vi "chooseXMLInstantiation.vi"(8 "error in (no error)":errorcluster, 10 "XMLin":string, 11 "TCSTcsCommand in":refnum<class "TCSTcsCommand.lvclass">) -> (0 "error out":errorcluster, 3 "TCSTcsCommand out":refnum<class "TCSTcsCommand.lvclass">)   [LabVIEW 2022 SP3, in "TCSDataDefinitions.lvlib" / "TCSCommand.lvlib" / "TCSTcsCommand.lvclass"]
uses:
  TCSTcsCommand.lvclass
  TCSCommand/commandInstantiation.ctl
  InstrumentSelect/InstrumentSelect.lvclass
  C:/Development/rimas/RIMAS/TCS/TCS_external_interfaces/TCSDataDefinitions/TCSCommand/TCSTcsCommand/TCSTcsCommand.lvclass
  TCSDebug/TCSDebug.lvclass
  M1Cover/M1Cover.lvclass
  OffsetCommands/ScienceTargetOffset/ScienceTargetOffset.lvclass
  OffsetCommands/GuideTargetOffset/GuideTargetOffset.lvclass
  OffsetCommands/WavefrontTargetOffset/WavefrontTargetOffset.lvclass
  OffsetCommands/ScienceTargetAbsorbOffset/ScienceTargetAbsorbOffset.lvclass
  OffsetCommands/GuideTargetAbsorbOffset/GuideTargetAbsorbOffset.lvclass
  OffsetCommands/WavefrontAbsorbOffset/WavefrontAbsorbOffset.lvclass
  OffsetCommands/ScienceTargetClearOffset/ScienceTargetClearOffset.lvclass
  OffsetCommands/GuideTargetClearOffset/GuideTargetClearOffset.lvclass
  OffsetCommands/WavefrontTargetClearOffset/WavefrontTargetClearOffset.lvclass
  OffsetCommands/ClearCollOffset/ClearCollOffset.lvclass
  OffsetCommands/CollOffset/CollOffset.lvclass
  OffsetCommands/RotOffset/RotOffset.lvclass
  POriginCommands/POrigin/POrigin.lvclass
  POriginCommands/POffset/POffset.lvclass
  POriginCommands/AbsorbPOrigin/AbsorbPOrigin.lvclass
  POriginCommands/ClearPOrigin/ClearPOrigin.lvclass
  AmLimit/AmLimit.lvclass
  SetAccessMode/SetOperatorAccessMode/SetOperatorAccessMode.lvclass
  SetAccessMode/SetEngineerAccessMode/SetEngineerAccessMode.lvclass
  StartUp/StartUp.lvclass
  ShutDown/ShutDown.lvclass
  GuiderCommands/Guide/Guide.lvclass
  GuiderCommands/GuideClear/GuideClear.lvclass
  GuiderCommands/GuideAutoclearState/GuideAutoclearState.lvclass
  PointingFileCommands/PointNew/PointNew.lvclass
  PointingFileCommands/PointAdd/PointAdd.lvclass
  TargetConfiguration/WavefrontTargetConfiguration/WavefrontTargetConfiguration.lvclass
  TargetConfiguration/GuideTargetConfiguration/GuideTargetConfiguration.lvclass
  TargetConfiguration/ScienceTargetConfiguration/ScienceTargetConfiguration.lvclass
  CableWrapCommands/RotCurrentWrap/RotCurrentWrap.lvclass
  CableWrapCommands/AzCurrentWrap/AzCurrentWrap.lvclass
  <vilib>/Utility/error.llb/Trim Whitespace.vi
  <vilib>/Utility/error.llb/Trim Whitespace One-Sided.vi
  <userlib>/Common/XML/XMLParser/XMLParser.lvclass
  TCSCommand.lvlib
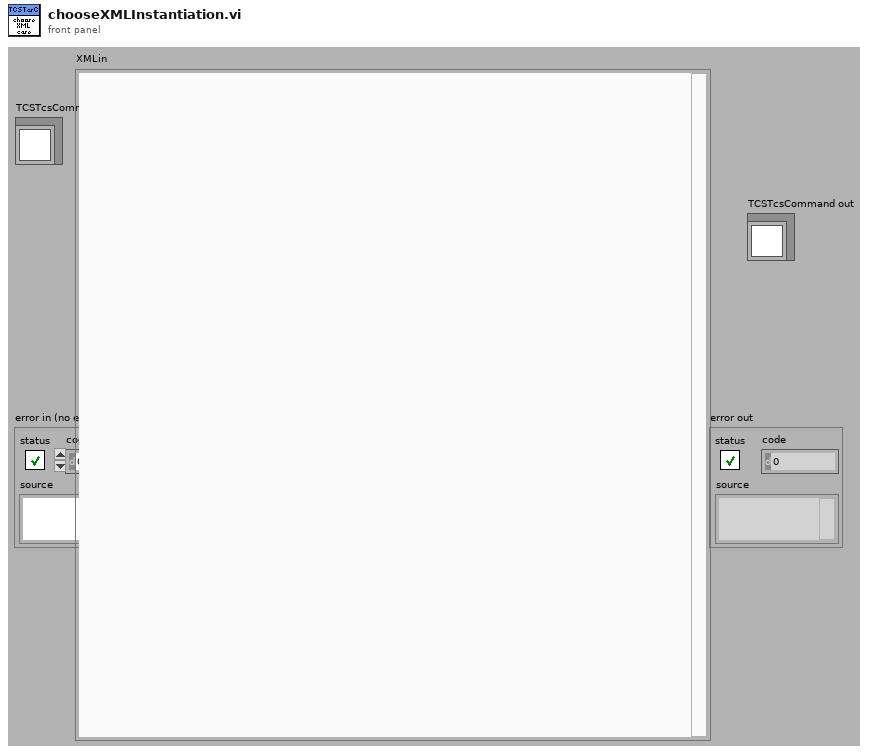
[diagram p1: front panel]
types:
  T1 = typedef "TCSDataDefinitions.lvlib/TCSCommand.lvlib/CommandInstantiation.ctl" = enum16{"focusSelect", "tcsDebug", "m1Cover", "scienceTargetOffset", "guideTargetOffset", "wavefrontTargetOffset", "scienceTargetAbsorbOffset", "guideTargetAbsorbOffset", "wavefrontTargetAbsorbOffset", "scienceTargetClearOffset", "guideTargetClearOffset", "wavefrontTargetClearOffset", "clearCollOffset", "collOffset", "rotOffset", "pOrigin", "pOffset", "absorbPOrigin", "clearPOrigin", "amLimit", "setOperatorAccessMode", "setEngineerAccessMode", "startUp", "shutDown", "guide", "guideClear", "guideAutoClearState", "pointNew", "pointAdd", "wavefrontTargetConfiguration", "guideTargetConfiguration", "scienceTargetConfiguration", "rotCurrentWrap", "azCurrentWrap"}
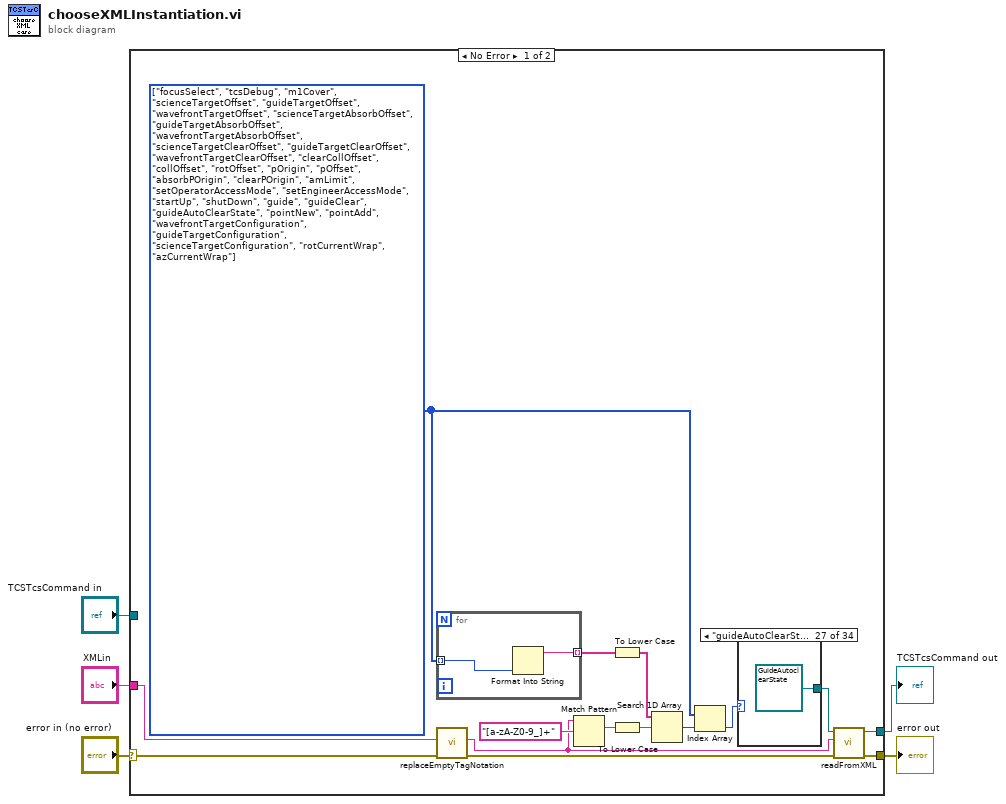
[diagram p0: block diagram]
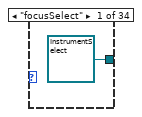
[diagram p2: hidden frame]
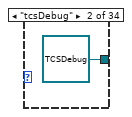
[diagram p3: hidden frame]
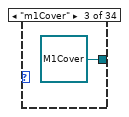
[diagram p4: hidden frame]
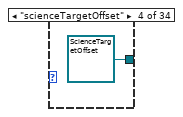
[diagram p5: hidden frame]
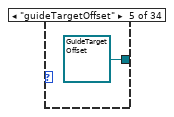
[diagram p6: hidden frame]
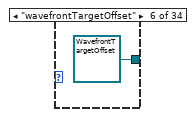
[diagram p7: hidden frame]
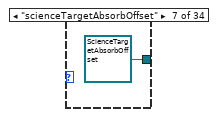
[diagram p8: hidden frame]
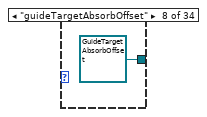
[diagram p9: hidden frame]
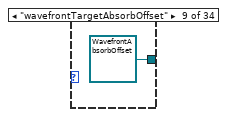
[diagram p10: hidden frame]
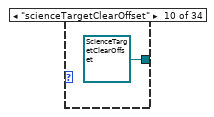
[diagram p11: hidden frame]
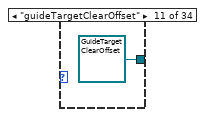
[diagram p12: hidden frame]
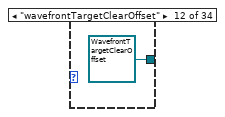
[diagram p13: hidden frame]
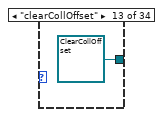
[diagram p14: hidden frame]
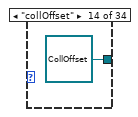
[diagram p15: hidden frame]
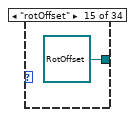
[diagram p16: hidden frame]
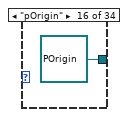
[diagram p17: hidden frame]
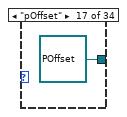
[diagram p18: hidden frame]
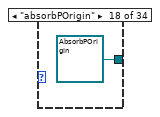
[diagram p19: hidden frame]
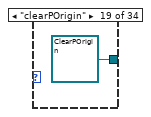
[diagram p20: hidden frame]
diagram:
  n1 = case shown="No Error" "error in (no error)" {
    selector: "error in (no error)" -> [w12 w58]
    tunnel: [w15 w58] -> w4
    tunnel: [w10 w57] -> w2
    tunnel: "TCSTcsCommand in" -> [_ w57]
    tunnel: "XMLin" -> [w14 _]
    frame No Error {
      w19 = T1[] [enum."focusSelect", enum."tcsDebug", enum."m1Cover", enum."scienceTargetOffset", enum."guideTargetOffset", enum."wavefrontTargetOffset", enum."scienceTargetAbsorbOffset", enum."guideTargetAbsorbOffset", enum."wavefrontTargetAbsorbOffset", enum."scienceTargetClearOffset", enum."guideTargetClearOffset", enum."wavefrontTargetClearOffset", enum."clearCollOffset", enum."collOffset", enum."rotOffset", enum."pOrigin", enum."pOffset", enum."absorbPOrigin", enum."clearPOrigin", enum."amLimit", enum."setOperatorAccessMode", enum."setEngineerAccessMode", enum."startUp", enum."shutDown", enum."guide", enum."guideClear", enum."guideAutoClearState", enum."pointNew", enum."pointAdd", enum."wavefrontTargetConfiguration", enum."guideTargetConfiguration", enum."scienceTargetConfiguration", enum."rotCurrentWrap", enum."azCurrentWrap"] items=["focusSelect", "tcsDebug", "m1Cover", "scienceTargetOffset", "guideTargetOffset", "wavefrontTargetOffset", "scienceTargetAbsorbOffset", "guideTargetAbsorbOffset", "wavefrontTargetAbsorbOffset", "scienceTargetClearOffset", "guideTargetClearOffset", "wavefrontTargetClearOffset", "clearCollOffset", "collOffset", "rotOffset", "pOrigin", "pOffset", "absorbPOrigin", "clearPOrigin", "amLimit", "setOperatorAccessMode", "setEngineerAccessMode", "startUp", "shutDown", "guide", "guideClear", "guideAutoClearState", "pointNew", "pointAdd", "wavefrontTargetConfiguration", "guideTargetConfiguration", "scienceTargetConfiguration", "rotCurrentWrap", "azCurrentWrap"]
      n2 = for {
        tunnel: w19 -> [w56] mode=indexing
        tunnel: [w55] -> w9 mode=indexing
        n3 = Format Into String(w56) -> (resulting string=w55:string)  [unwired: 3 in, 1 out]
      }
      n4 = call <userlib>:"replaceEmptyTagNotation.vi"("error in (no error)"=w12, "XML in"=w14) -> ("error out"=w11:errorcluster, "XML out"=w13:string)  [unwired: 7 in, 1 out]
      n5 = Match Pattern(string=w13, regular expression="[a-zA-Z0-9_]+") -> (match substring=w7:string)  [unwired: 1 in, 3 out]
      n6 = To Lower Case(string=w9) -> (all lower case string=w8:string[])
      n7 = To Lower Case(string=w7) -> (all lower case string=w6:string)
      n8 = Search 1D Array(1D array=w8, element=w6) -> (index of element=w18:i32)  [unwired: 1 in]
      n9 = Index Array(array=w19, index=w18) -> (element=w17:T1)
      n10 = case shown="\"guideAutoClearState\"" w17 {
        tunnel: [refnum<class "InstrumentSelect.lvclass"> refnum ("FocusSelect.lvclass") refnum<class "TCSDebug.lvclass"> refnum ("TCSDebug.lvclass") refnum<class "M1Cover.lvclass"> refnum ("M1Cover.lvclass") refnum<class "ScienceTargetOffset.lvclass"> refnum ("ScienceTargetOffset.lvclass") refnum<class "GuideTargetOffset.lvclass"> refnum ("GuideTargetOffset.lvclass") refnum<class "WavefrontTargetOffset.lvclass"> refnum ("WavefrontTargetOffset.lvclass") refnum<class "ScienceTargetAbsorbOffset.lvclass"> refnum ("ScienceTargetAbsorbOffset.lvclass") refnum<class "GuideTargetAbsorbOffset.lvclass"> refnum ("GuideTargetAbsorbOffset.lvclass") refnum<class "WavefrontAbsorbOffset.lvclass"> refnum ("WavefrontAbsorbOffset.lvclass") refnum<class "ScienceTargetClearOffset.lvclass"> refnum ("ScienceTargetClearOffset.lvclass") refnum<class "GuideTargetClearOffset.lvclass"> refnum ("GuideTargetClearOffset.lvclass") refnum<class "WavefrontTargetClearOffset.lvclass"> refnum ("WavefrontTargetClearOffset.lvclass") refnum<class "ClearCollOffset.lvclass"> refnum ("ClearCollOffset.lvclass") refnum<class "CollOffset.lvclass"> refnum ("CollOffset.lvclass") refnum<class "RotOffset.lvclass"> refnum ("RotOffset.lvclass") refnum<class "POrigin.lvclass"> refnum ("POrigin.lvclass") refnum<class "POffset.lvclass"> refnum ("POffset.lvclass") refnum<class "AbsorbPOrigin.lvclass"> refnum ("AbsorbPOrigin.lvclass") refnum<class "ClearPOrigin.lvclass"> refnum ("ClearPOrigin.lvclass") refnum<class "AmLimit.lvclass"> refnum ("AmLimit.lvclass") refnum<class "SetOperatorAccessMode.lvclass"> refnum ("SetOperatorAccessMode.lvclass") refnum<class "SetEngineerAccessMode.lvclass"> refnum ("SetEngineerAccessMode.lvclass") refnum<class "StartUp.lvclass"> refnum ("StartUp.lvclass") refnum<class "ShutDown.lvclass"> refnum ("ShutDown.lvclass") refnum<class "Guide.lvclass"> refnum ("Guide.lvclass") refnum<class "GuideClear.lvclass"> refnum ("GuideClear.lvclass") refnum<class "GuideAutoclearState.lvclass"> refnum ("GuideAutoclearState.lvclass") refnum<class "PointNew.lvclass"> refnum ("PointNew.lvclass") refnum<class "PointAdd.lvclass"> refnum ("PointAdd.lvclass") refnum<class "WavefrontTargetConfiguration.lvclass"> refnum ("WavefrontTargetConfiguration.lvclass") refnum<class "GuideTargetConfiguration.lvclass"> refnum ("GuideTargetConfiguration.lvclass") refnum<class "ScienceTargetConfiguration.lvclass"> refnum ("ScienceTargetConfiguration.lvclass") refnum<class "RotCurrentWrap.lvclass"> refnum ("RotCurrentWrap.lvclass") refnum<class "AzCurrentWrap.lvclass"> refnum ("AzCurrentWrap.lvclass")] -> w16
        frame "focusSelect" {
        }
        frame "tcsDebug" {
        }
        frame "m1Cover" {
        }
        frame "scienceTargetOffset" {
        }
        frame "guideTargetOffset" {
        }
        frame "wavefrontTargetOffset" {
        }
        frame "scienceTargetAbsorbOffset" {
        }
        frame "guideTargetAbsorbOffset" {
        }
        frame "wavefrontTargetAbsorbOffset" {
        }
        frame "scienceTargetClearOffset" {
        }
        frame "guideTargetClearOffset" {
        }
        frame "wavefrontTargetClearOffset" {
        }
        frame "clearCollOffset" {
        }
        frame "collOffset" {
        }
        frame "rotOffset" {
        }
        frame "pOrigin" {
        }
        frame "pOffset" {
        }
        frame "absorbPOrigin" {
        }
        frame "clearPOrigin" {
        }
        frame "amLimit" {
        }
        frame "setOperatorAccessMode" {
        }
        frame "setEngineerAccessMode" {
        }
        frame "startUp" {
        }
        frame "shutDown" {
        }
        frame "guide" {
        }
        frame "guideClear" {
        }
        frame "guideAutoClearState" {
        }
        frame "pointNew" {
        }
        frame "pointAdd" {
        }
        frame "wavefrontTargetConfiguration" {
        }
        frame "guideTargetConfiguration" {
        }
        frame "scienceTargetConfiguration" {
        }
        frame "rotCurrentWrap" {
        }
        frame "azCurrentWrap" {
        }
      }
      n11 = call-dynamic "readFromXML.vi"("error in (no error)"=w11, "XMLin"=w13, "TCSTcsCommand in"=w16) -> ("error out"=w15:errorcluster, "TCSTcsCommand out"=w10:refnum<class "TCSTcsCommand.lvclass">)  [unwired: 7 in]
    }
    frame Error {
    }
  }
  "error out" <- w4
  "TCSTcsCommand out" <- w2
